vi "Close Log.vi"(0 "reference in":refnum<class "Logger.lvclass">, 2 "timeout in ms (-1)":i32=-1, 5 "Error In":errorcluster) -> (14 "reference out":refnum<class "Logger.lvclass">, 16 "log file path":path, 19 "Error Out":errorcluster)   [LabVIEW 2023, in "Logger.lvclass"]
uses:
  Logger.lvclass
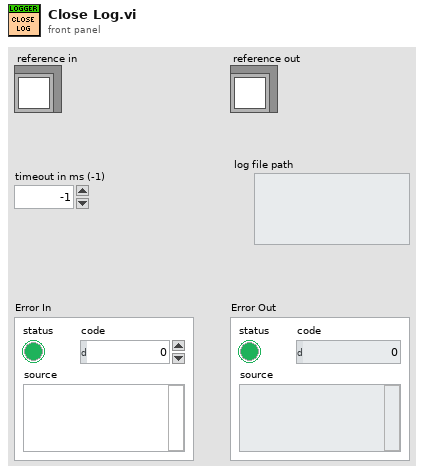
[diagram p1: front panel]
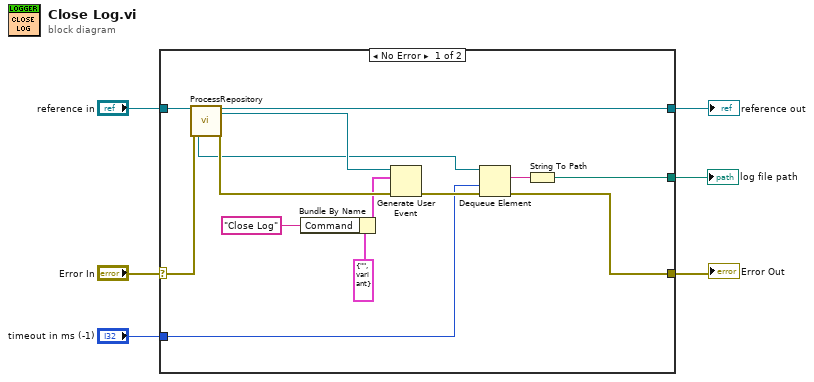
[diagram p0: block diagram]
diagram:
  n1 = case shown="No Error" "Error In" {
    selector: "Error In" -> [w20 w22]
    tunnel: [w14 w22] -> w5
    tunnel: [w18 w21] -> w3
    tunnel: "reference in" -> [w19 w21]
    tunnel: "timeout in ms (-1)" -> [w9 _]
    tunnel: [w7 _] -> w1
    frame No Error {
      n2 = call "ProcessRepository.vi"("reference in"=w19, "Error In"=w20) -> ("QueueFromProcess"=w11:refnum<queue>, "reference out"=w18:refnum<class "Logger.lvclass">, "EventsToProcess"=w17:refnum<user-event>, "Error Out"=w15:errorcluster)  [unwired: 10 in, 4 out]
      n3 = Bundle By Name(cluster=cluster{"Command":string, "Data":variant} {"Command"="", "Data"=variant} ("MessageToProcess"), "Command"="Close Log") -> (w12:cluster{"Command":string, "Data":variant})
      n4 = Generate User Event(user event=w17, event data cluster=w12, error in=w15) -> (error out=w16:errorcluster)  [unwired: 1 in, 1 out]
      n5 = Dequeue Element(queue=w11, timeout in ms (-1)=w9, error in (no error)=w16) -> (element=w8:string, error out=w14:errorcluster)  [unwired: 2 out]
      n6 = String To Path(string=w8) -> (path=w7:path)
    }
    frame Error {
    }
  }
  "Error Out" <- w5
  "reference out" <- w3
  "log file path" <- w1
